vi "Consumer.vi"(8 "error in (no error)":errorcluster, 9 "Data":variant, 10 "Case ID":string, 11 "Error Manager in":refnum<class "Error Manager.lvclass">) -> (0 "error out":errorcluster, 3 "Error Manager out":refnum<class "Error Manager.lvclass">)   [LabVIEW 2026, in "TALOS.lvlib" / "Error Manager.lvlib" / "Error Manager.lvclass"]
uses:
  Error Manager.lvclass
  Error Manager Consumer Case Selector.ctl
  Error Info.ctl
  Ancestor/Ancestor/Ancestor.lvclass/Ancestor.ctl
  Support VIs/Generate Error.vi
  FGV/Error Memory/Get Error Description.vi
  Support VIs/Get PC name.vi
  Ancestor/Ancestor/Read ID.vi
  Support VIs/Get Class Name.vi
  <vilib>/Utility/error.llb/Clear Errors.vi
  FGV/Error Memory/Error Memory Core.vi
  <vilib>/AdvancedString/Delimited String to 1D String Array.vi
  <vilib>/AdvancedString/Delimited String to 1D String Array (string).vi
  Support VIs/Circus Root Path.vi
  FGV/Error Memory/Error Crt Lvl checker.vi
  FGV/Error Memory/Error Memory Core.vi/40c8088d-b597-4017-91af-faa98e00292e.vi
  FGV/Error Memory/Error Memory Core.vi/d4a3ab98-063c-4e44-b43d-fbdcfe6c2be2.vi
  Support VIs/Global Memory.vi
  <vilib>/Utility/LVClass/Get LV Class Name.vi
  Support VIs/Is in Packed Library.vi
  Support VIs/TALOS Root path.vi
  Support VIs/Read CSV worksheet.vi
  Support VIs/Global Constants.vi
  <vilib>/Utility/error.llb/General Error Handler.vi
  Support VIs/Error Log.vi
  Ancestor/Ancestor/Ancestor.lvclass
  <vilib>/Comparison/Equal/Equal Functor/Equal Functor.lvclass
  Father of all uServices/Father of all uServices/Father of all uServices.lvclass
  TALOS.lvlib
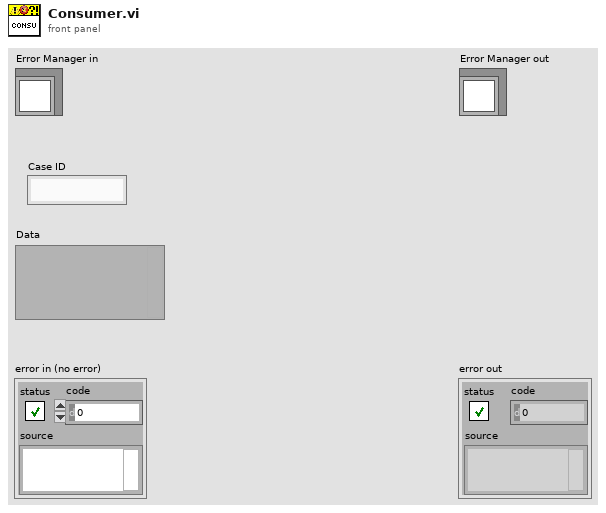
[diagram p1: front panel]
types:
  T1 = typedef "TALOS.lvlib/Error Manager.lvlib/Error Manager.lvclass/Error Manager Consumer Case Selector.ctl" = enum16{"Digest Error", "Dismiss Error", "Dismiss All", "Show Error Details", "Filter out Errors", "Clear Filters", "Check Distributed Mngr Status"}
  T2 = typedef "TALOS.lvlib/Error Manager.lvlib/Error Manager.lvclass/Error Info.ctl" = cluster{"error out":errorcluster, "Time Stamp":timestamp, "Machine Name":string, "GUID":string}
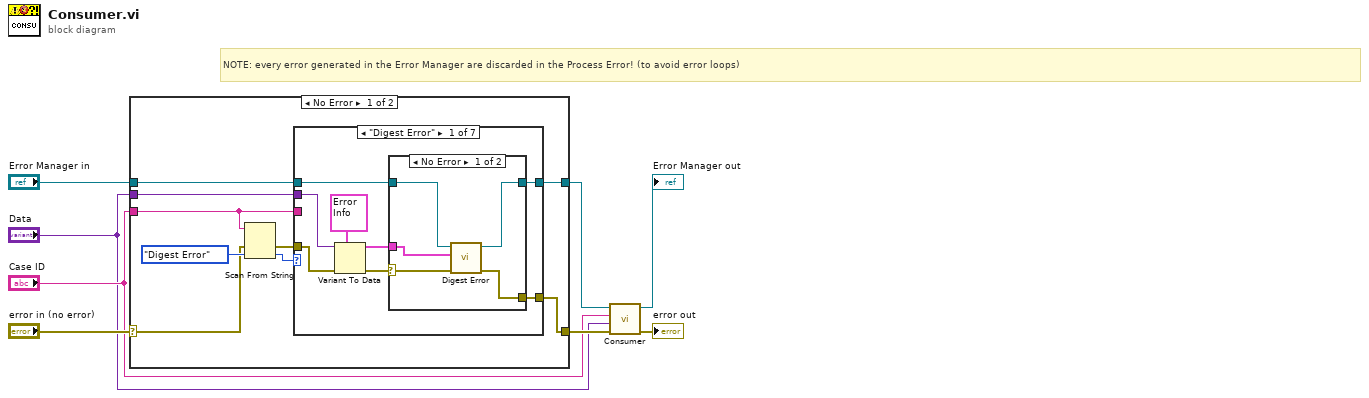
[diagram p0: block diagram]
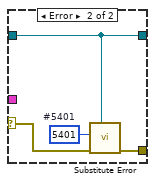
[diagram p2: hidden frame]
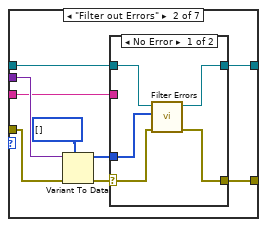
[diagram p3: hidden frame]
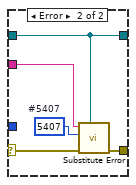
[diagram p4: hidden frame]
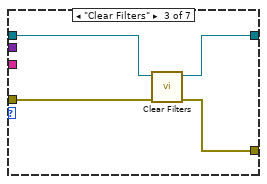
[diagram p5: hidden frame]
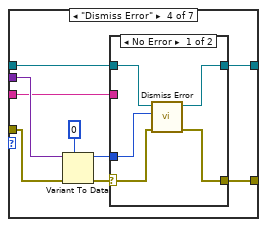
[diagram p6: hidden frame]
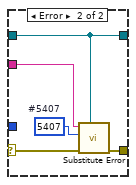
[diagram p7: hidden frame]
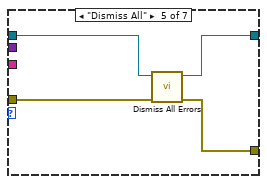
[diagram p8: hidden frame]
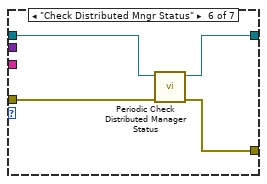
[diagram p9: hidden frame]
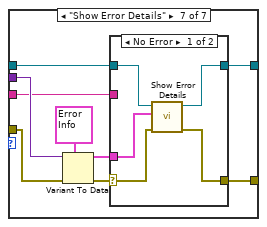
[diagram p10: hidden frame]
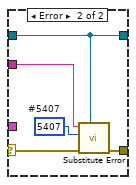
[diagram p11: hidden frame]
diagram:
  # "NOTE: every error generated in the Error Manager are discarded in the Process Error! (to avoid error loops)"
  n1 = case shown="No Error" "error in (no error)" {
    selector: "error in (no error)" -> [w13 w104]
    tunnel: [w10 w105] -> w7
    tunnel: "Error Manager in" -> [w17 w105]
    tunnel: [w15 w104] -> w8
    tunnel: "Case ID" -> [w9 _]
    tunnel: "Data" -> [w16 _]
    frame No Error {
      n2 = Scan From String(input string=w9, error in=w13, default 1=Error_Manager_Consumer_Case_Selector."Digest Error" ("ErrMgr Case Selector")) -> (error out=w12:errorcluster, output 1=w11:T1)  [unwired: 2 in, 2 out]
      n3 = case shown="\"Digest Error\"" w11 {
        tunnel: w17 -> [w23 w43 w57 w66 w80 w84 w93]
        tunnel: w16 -> [w21 w38 _ w61 _ _ w89]
        tunnel: [w25 w42 w56 w65 w79 w82 w92] -> w15
        tunnel: w12 -> [w22 w39 w54 w62 w77 w81 w90]
        tunnel: [w24 w41 w55 w64 w78 w83 w91] -> w10
        tunnel: w9 -> [_ w35 _ w58 _ _ w86]
        frame "Digest Error" {
          n4 = Variant To Data(error in=w22, type=T2 {"error out"={"status"=FALSE, "code"=0, "source"=""}, "Time Stamp"=timestamp(0 s since 1904-01-01), "Machine Name"="", "GUID"=""} ("Array"), Variant=w21) -> (data=w18:T2, error out=w19:errorcluster)
          n5 = case shown="No Error" w19 {
            selector: w19 -> [w27 w33]
            tunnel: [w30 w32] -> w25
            tunnel: [w29 w31] -> w24
            tunnel: w23 -> [w28 w31]
            tunnel: w18 -> [w26 _]
            frame No Error {
              n6 = call-dynamic "Digest Error.vi"("error in (no error)"=w27, "TALOS Error In"=w26, "Error Manager in"=w28) -> ("error out"=w30:errorcluster, "Error Manager out"=w29:refnum<class "Error Manager.lvclass">)  [unwired: 7 in]
            }
            frame Error {
              w34 = 5401  # #5401
              n7 = call "Substitute Error.vi"("LabVIEW Object"=w31, "error in (no error)"=w33, "Error Code"=w34) -> ("error out"=w32:errorcluster)  [unwired: 8 in]
            }
          }
        }
        frame "Filter out Errors" {
          n8 = Variant To Data(error in=w39, type=i32[] [], Variant=w38) -> (data=w36:i32[], error out=w37:errorcluster)
          n9 = case shown="No Error" w37 {
            selector: w37 -> [w44 w52]
            tunnel: w43 -> [w48 w50]
            tunnel: [w47 w51] -> w42
            tunnel: [w46 w50] -> w41
            tunnel: w36 -> [w45 _]
            tunnel: w35 -> [_ w49]
            frame No Error {
              n10 = call-dynamic "Filter Errors.vi"("error in (no error)"=w44, "Errors to filter"=w45, "Error Manager in"=w48) -> ("error out"=w47:errorcluster, "Error Manager out"=w46:refnum<class "Error Manager.lvclass">)  [unwired: 6 in, 1 out]
            }
            frame Error {
              w53 = 5407  # #5407
              n11 = call "Substitute Error.vi"("LabVIEW Object"=w50, "error in (no error)"=w52, "Error Code"=w53, "Optional String"=w49) -> ("error out"=w51:errorcluster)  [unwired: 7 in]
            }
          }
        }
        frame "Clear Filters" {
          n12 = call-dynamic "Clear Filters.vi"("error in (no error)"=w54, "Error Manager in"=w57) -> ("error out"=w56:errorcluster, "Error Manager out"=w55:refnum<class "Error Manager.lvclass">)  [unwired: 7 in, 1 out]
        }
        frame "Dismiss Error" {
          n13 = Variant To Data(error in=w62, type=0, Variant=w61) -> (data=w59:i32, error out=w60:errorcluster)
          n14 = case shown="No Error" w60 {
            selector: w60 -> [w67 w75]
            tunnel: w66 -> [w71 w73]
            tunnel: [w70 w74] -> w65
            tunnel: [w69 w73] -> w64
            tunnel: w59 -> [w68 _]
            tunnel: w58 -> [_ w72]
            frame No Error {
              n15 = call-dynamic "Dismiss Error.vi"("error in (no error)"=w67, "Select Error"=w68, "Error Manager in"=w71) -> ("error out"=w70:errorcluster, "Error Manager out"=w69:refnum<class "Error Manager.lvclass">)  [unwired: 7 in]
            }
            frame Error {
              w76 = 5407  # #5407
              n16 = call "Substitute Error.vi"("LabVIEW Object"=w73, "error in (no error)"=w75, "Error Code"=w76, "Optional String"=w72) -> ("error out"=w74:errorcluster)  [unwired: 7 in]
            }
          }
        }
        frame "Dismiss All" {
          n17 = call-dynamic "Dismiss All Errors.vi"("error in (no error)"=w77, "Error Manager in"=w80) -> ("error out"=w79:errorcluster, "Error Manager out"=w78:refnum<class "Error Manager.lvclass">)  [unwired: 8 in]
        }
        frame "Check Distributed Mngr Status" {
          n18 = call-dynamic "Periodic Check Distributed Manager Status.vi"("error in (no error)"=w81, "Error Manager in"=w84) -> ("error out"=w82:errorcluster, "Error Manager out"=w83:refnum<class "Error Manager.lvclass">)  [unwired: 8 in]
        }
        frame "Show Error Details" {
          n19 = Variant To Data(error in=w90, type=T2 {"error out"={"status"=FALSE, "code"=0, "source"=""}, "Time Stamp"=timestamp(0 s since 1904-01-01), "Machine Name"="", "GUID"=""} ("Error Info"), Variant=w89) -> (data=w87:T2, error out=w88:errorcluster)
          n20 = case shown="No Error" w88 {
            selector: w88 -> [w94 w102]
            tunnel: w93 -> [w98 w100]
            tunnel: [w97 w101] -> w92
            tunnel: [w96 w100] -> w91
            tunnel: w87 -> [w95 _]
            tunnel: w86 -> [_ w99]
            frame No Error {
              n21 = call-dynamic "Show Error Details.vi"("error in (no error)"=w94, "Error Info"=w95, "Error Manager in"=w98) -> ("error out"=w97:errorcluster, "Error Manager out"=w96:refnum<class "Error Manager.lvclass">)  [unwired: 7 in]
            }
            frame Error {
              w103 = 5407  # #5407
              n22 = call "Substitute Error.vi"("LabVIEW Object"=w100, "error in (no error)"=w102, "Error Code"=w103, "Optional String"=w99) -> ("error out"=w101:errorcluster)  [unwired: 7 in]
            }
          }
        }
      }
    }
    frame Error {
    }
  }
  n23 = call-parent "Consumer.vi"("error in (no error)"=w8, "Data"="Data", "Case ID"="Case ID", "uService Template in"=w7) -> ("error out"=→"error out":errorcluster, "uService Template out"=→"Error Manager out":refnum<class "Error Manager.lvclass">)  [unwired: 6 in]
